vi "Waveform - Get Final Time and Duration.vi"() -> ()   [LabVIEW 2023]
doc: "Shows how to get the final time and duration of the waveform."
uses:
  <vilib>/Waveform/WDTOps.llb/Get Final Time Value.vi
  <vilib>/Waveform/WDTOps.llb/WDT Get Final Time Value DBL.vi
  <vilib>/Waveform/WDTOps.llb/Waveform Duration.vi
  <vilib>/Waveform/WDTOps.llb/WDT Waveform Duration DBL.vi
  <vilib>/Waveform/WDTOps.llb/WDT Number of Waveform Samples DBL.vi
panel:
  out "Waveform":waveform(dbl)(graph)
  out "Number of Samples":i32
  out "Duration":dbl format="%.2f"
  out "Final Time":timestamp
  # "Overview: Demonstrates the use of multiple Waveform VIs to obtain information about a waveform.\nInstructions:\nRun the VI. The Final Time, Duration, and Number of Samples of the waveform will be displayed."
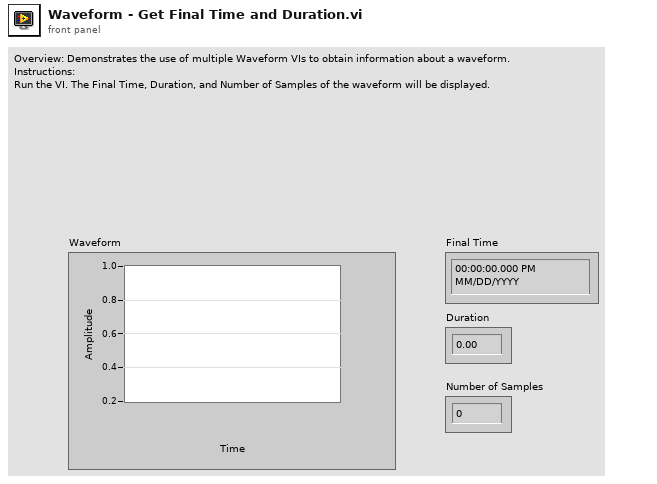
[diagram p1: front panel]
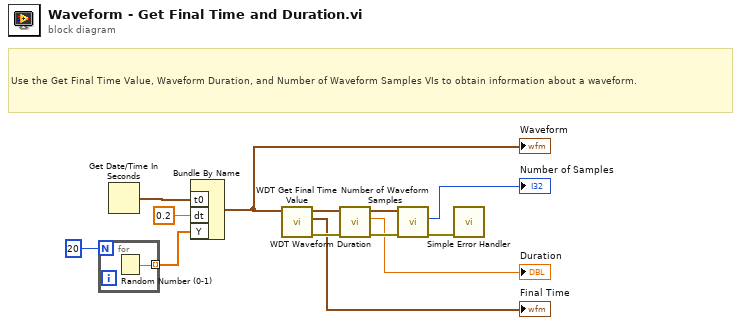
[diagram p0: block diagram]
diagram:
  # "Use the Get Final Time Value, Waveform Duration, and Number of Waveform Samples VIs to obtain information about a waveform."
  n1 = for {
    N: 20 -> [_]
    tunnel: [w14] -> w4 mode=indexing
    n2 = Random Number (0-1)() -> (number: 0 to 1=w14:dbl)
  }
  n3 = Get Date/Time In Seconds() -> (seconds since 1Jan1904=w3:timestamp)
  n4 = Bundle By Name("t0"=w3, "dt"=0.2, "Y"=w4) -> (w6:waveform(dbl))  [unwired: 1 in]
  "Waveform" <- w6
  n5 = call-poly "WDT Get Final Time Value.vi"("waveform in"=w6) -> ("error out"=w11:errorcluster, "tf"=→"Final Time":timestamp, "waveform out"=w13:waveform(dbl))  [unwired: 8 in]
  n6 = call-poly "WDT Waveform Duration.vi"("error in (no error)"=w11, "waveform in"=w13) -> ("error out"=w10:errorcluster, "duration"=→"Duration":dbl, "waveform out"=w12:waveform(dbl))  [unwired: 7 in]
  n7 = call-poly <vilib>:"Number of Waveform Samples.vi"("error in (no error)"=w10, "waveform in"=w12) -> ("error out"=w1:errorcluster, "number of samples"=→"Number of Samples":i32)  [unwired: 7 in, 1 out]
  n8 = call <vilib>:"Simple Error Handler.vi"("error in (no error)"=w1) -> ()  [unwired: 4 in, 5 out]
